vi "Draw.vi"(8 "Error In":errorcluster, 11 "Display Element In":refnum<class "Display Element.lvclass">) -> (0 "Error Out":errorcluster, 2 "Element To Display":T1[](array[typedef]), 3 "Display Element Out":refnum<class "Display Element.lvclass">)   [LabVIEW 2019, in "Display Element.lvclass"]
uses:
  Display Element.lvclass
  Controls/Vector.ctl
  Controls/Pixel.ctl
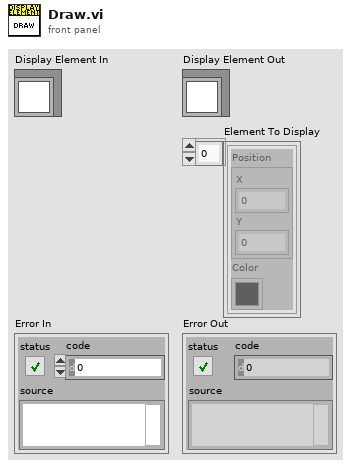
[diagram p1: front panel]
types:
  T1 = typedef "Display Element.lvclass/Pixel.ctl" = cluster{"Position":T2, "Color":u32}
  T2 = typedef "Display Element.lvclass/Vector.ctl" = cluster{"X":i32, "Y":i32}
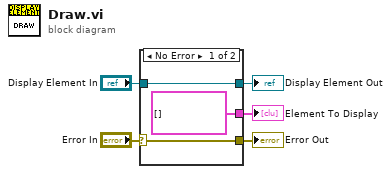
[diagram p0: block diagram]
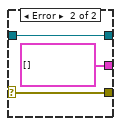
[diagram p2: hidden frame]
diagram:
  n1 = case shown="No Error" "Error In" {
    selector: "Error In" -> [w8 w10]
    tunnel: "Display Element In" -> [w7 w11]
    tunnel: [w8 w10] -> w3
    tunnel: [w7 w11] -> w2
    tunnel: [T1[] [] T1[] []] -> w1
    frame No Error {
    }
    frame Error {
    }
  }
  "Display Element Out" <- w2
  "Error Out" <- w3
  "Element To Display" <- w1
